vi "Generate File paths.vi"(8 "error in":errorcluster) -> (0 "error out":errorcluster, 1 "Project path":path, 2 ".ini path":path)   [LabVIEW 2011]
doc: "This .vi generates the base path, .ini paths, and dynamically called .vi's based off of the project file (project file searched for) and sets these in a filepath global. The dynamically called .vi's are checked that they exist.\n\nThis subvi can also be used in other top level Quartz apps. It only runs on first call, so it can be safely repeatedly called, in any vi within the project."
uses:
  Filepaths global.vi
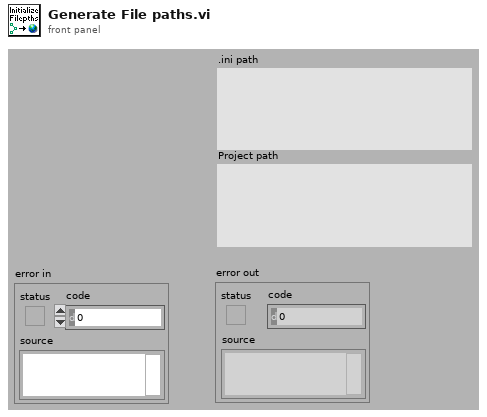
[diagram p1: front panel]
types:
  T1 = typedef "ProjectName enum.ctl" = enum16{"V-SIM", "SPIM", "TEMca2", "undefined"}
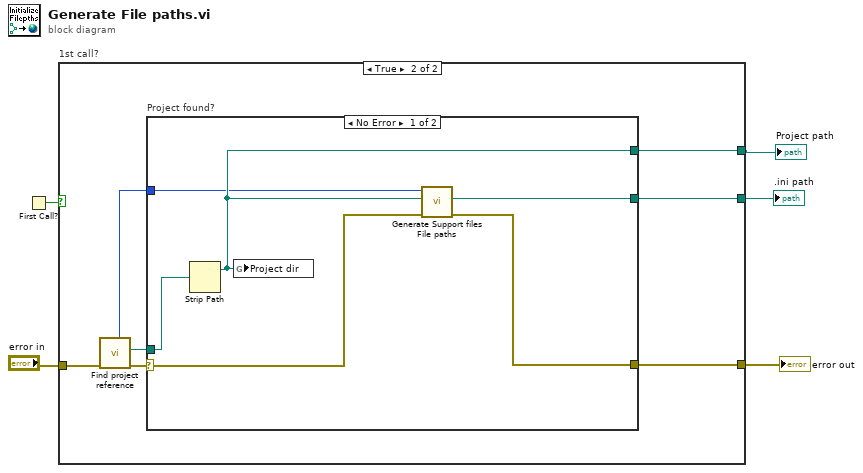
[diagram p0: block diagram]
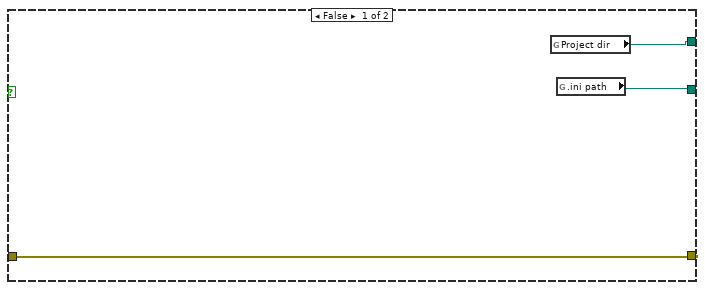
[diagram p2: hidden frame]
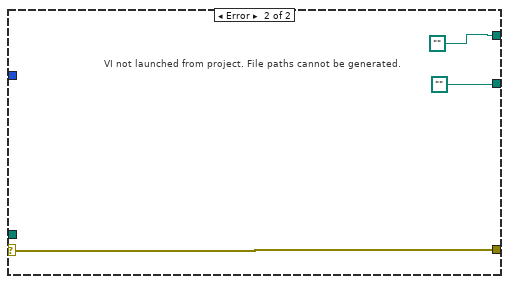
[diagram p3: hidden frame]
diagram:
  n1 = First Call?() -> (First Call?: T/F=w3:bool)
  n2 = case "1st call?" shown="True" w3 {
    tunnel: [w8 w11] -> w5
    tunnel: "error in" -> [w8 w14]
    tunnel: [w7 w13] -> w2
    tunnel: [w6 w12] -> w1
    frame False {
      n3 = global read "Filepaths global.vi" "Project dir"() -> (w6:path)
      n4 = global read "Filepaths global.vi" ".ini path"() -> (w7:path)
    }
    frame True {
      n5 = call "Find project reference.vi"("error in"=w14) -> ("ProjectName"=w10:T1, ".lvproj Filepath"=w15:path, "error out"=w9:errorcluster)  [unwired: 5 out]
      n6 = case "Project found?" shown="No Error" w9 {
        selector: w9 -> [w16 w22]
        tunnel: w15 -> [w20 _]
        tunnel: [w18 w22] -> w11
        tunnel: [w21 path ""] -> w13
        tunnel: [w19 path ""] -> w12
        tunnel: w10 -> [w17 _]
        frame No Error {
          n7 = Strip Path(path=w20) -> (stripped path=w19:path)  [unwired: 1 out]
          n8 = global write "Filepaths global.vi" "Project dir"(w19) -> ()
          n9 = call "Generate Support files File paths.vi"("error in"=w16, "base path"=w19, "ProjectName"=w17) -> ("error out"=w18:errorcluster, ".ini path"=w21:path)  [unwired: 3 out]
        }
        frame Error {
          # "VI not launched from project. File paths cannot be generated."
        }
      }
    }
  }
  "error out" <- w5
  ".ini path" <- w2
  "Project path" <- w1
